vi "SpielBeendet.vi"() -> ()   [LabVIEW 2017]
panel:
  in  "Boolesch":bool
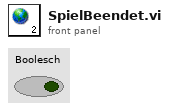
[diagram p1: front panel]
diagram:
